vi "test_SetLogLevel_SetDebug_EventLogged.vi"(8 "error in (no error)":errorcluster, 11 "TestCase in":refnum<class "TestDataSink.lvclass">) -> (0 "error out":errorcluster, 3 "TestCase out":refnum<class "TestDataSink.lvclass">)   [LabVIEW 2017, in "TestDataSink.lvclass"]
uses:
  TestDataSink.lvclass
  Source/Composed Log/Types/Log Level.ctl
  Source/LVQueue Sink/LVQueue Sink.lvclass/LVQueue Sink.ctl
  Source/Composed Log/LoggerReference/LoggerReference.lvclass/LoggerReference.ctl
  Source/Composed Log/Log Sink/Log Sink.lvclass/Log Sink.ctl
  7e94cd01-c0ee-42ed-b087-4c2160652887.vi
  7e94cd01-c0ee-42ed-b087-4c2160652887.vi/e6a5d2d2-facc-43d0-9f34-28763a163c9b.vi
  Source/Composed Log/LoggerReference/Return Aggregate Queues.vi
  Source/Composed Log/LoggerReference/Add Aggregate Log.vi
  7e94cd01-c0ee-42ed-b087-4c2160652887.vi/e6a5d2d2-facc-43d0-9f34-28763a163c9b.vi/21c004db-7efd-4755-bf90-e0fdfa4dea43.vi
  Source/Composed Log/LoggerReference/Log.vi
  Source/Composed Log/LoggerReference/Send Add Sink.vi
  Source/Composed Log/LoggerReference/Remove Stale Logs.vi
  Source/LVQueue Sink/LVQueue Sink.lvclass
  C:/CS/Internal/LabVIEW/Logger/Source/Composed Log/Log Sink/Log Sink.lvclass
  Source/Composed Log/Application Logger/Launch Worker Loop.vi
  Source/Composed Log/LoggerReference/Initialize Logger Instance.vi
  Source/Composed Log/Singleton Event Log/Logger Queue FGV.vi
  Source/Composed Log/IErrorFormat/IErrorFormat.lvclass
  Source/Composed Log/LoggerReference/LoggerReference.lvclass
  Source/Composed Log/Log Sink/Log Sink.lvclass
  <vilib>/addons/_JKI Toolkits/VI Tester/TestCase.llb/TestCase.lvclass
  Source/Composed Log/Singleton Event Log/Singleton Event Log.lvlib
  Source/Composed Log/Composed Log.lvlib
  C:/Program Files (x86)/National Instruments/LabVIEW 2017/vi.lib/addons/_JKI Toolkits/VI Tester/TestCase.llb/TestCase.lvclass
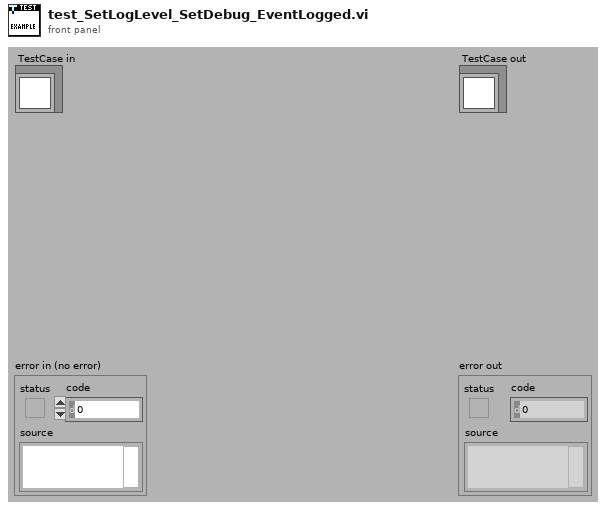
[diagram p1: front panel]
types:
  T1 = typedef "Composed Log.lvlib/Log Level.ctl" = enum16{"Debug", "Info", "Warning", "Error", "Critical"}
  T2 = typedef "Composed Log.lvlib/Log Packet.ctl" = cluster{"Data To Log":string, "Source":string, "Event Level":T1, "Event Time":timestamp}
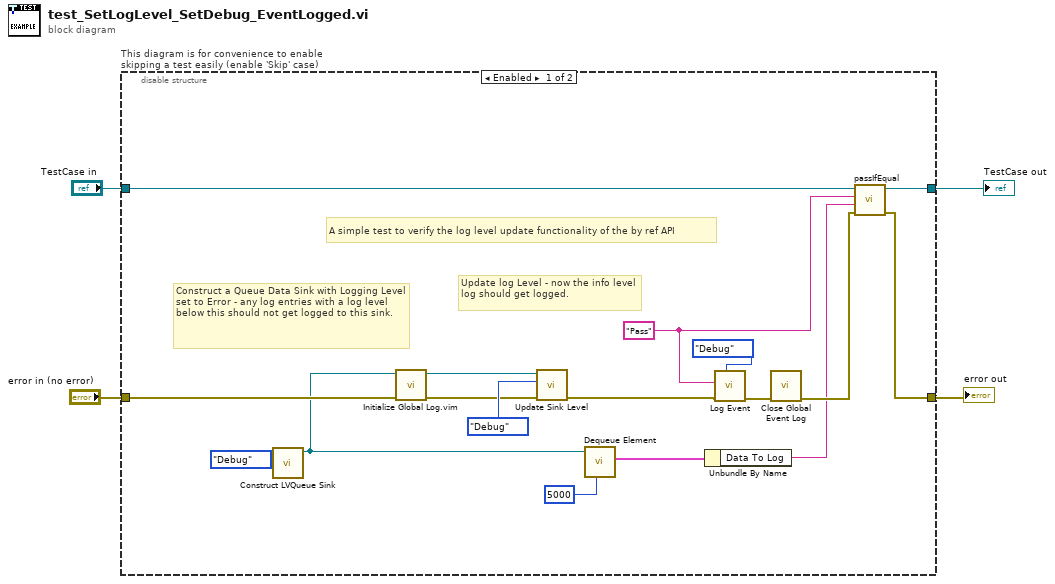
[diagram p0: block diagram]
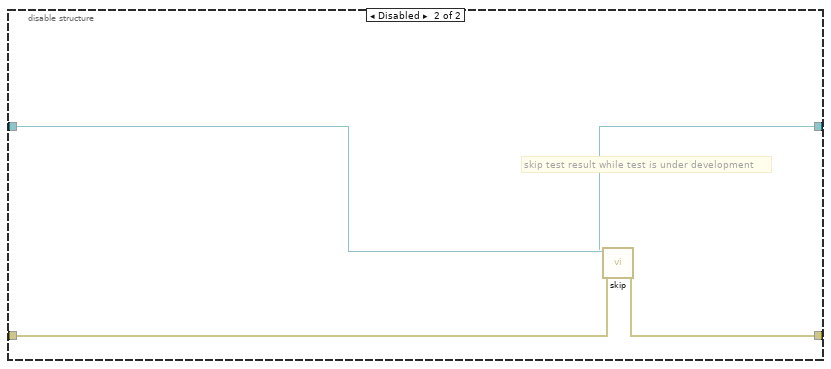
[diagram p2: hidden frame]
diagram:
  n1 = disable-structure "This diagram is for convenience to enable skipping a test easily (enable 'Skip' case)" shown="Enabled" {
    disable-tunnel: "TestCase in" -> [w18 w25]
    disable-tunnel: [w20 w23] -> w1
    disable-tunnel: [w19 w24] -> w3
    disable-tunnel: "error in (no error)" -> [w21 w22]
    frame Enabled {
      w6 = "Pass" ("Data To Log")
      # "Update log Level - now the info level log should get logged."
      # "A simple test to verify the log level update functionality of the by ref API"
      # "Construct a Queue Data Sink with Logging Level set to Error - any log entries with a log level below this should not get logged to this sink."
      n2 = call "Construct LVQueue Sink.vi"("LogLevel"=Log_Level."Debug") -> ("LVQueue Sink out"=w17:refnum<class "LVQueue Sink.lvclass">)  [unwired: 9 in, 1 out]
      n3 = call "Initialize Global Log.vim"("error in (no error)"=w21, "Log Sink(s)"=w17) -> ("error out"=w9:errorcluster, "Log Sink Reference(s)"=w15:refnum<data-value>)  [unwired: 8 in]
      n4 = call "Update Sink Level.vi"("error in (no error)"=w9, "LogLevel"=Log_Level."Debug", "Log Sink"=w15) -> ("error out"=w8:errorcluster)  [unwired: 8 in]
      n5 = call "Dequeue Element.vi"("timeout in ms (-1)"=5000, "LVQueue Sink in"=w17) -> ("Log Packet"=w12:T2)  [unwired: 6 in, 3 out]
      n6 = Unbundle By Name(w12) -> ("Data To Log"=w11:string)
      n7 = call "Log Event.vi"("Event Level"=Log_Level."Debug", "error in (no error)"=w8, "Data To Log"=w6) -> ("error out"=w7:errorcluster)  [unwired: 8 in]
      n8 = call "Close Global Event Log.vi"("error in (no error)"=w7) -> ("error out"=w13:errorcluster)  [unwired: 10 in]
      n9 = call-dynamic "passIfEqual.vi"("error in (no error)"=w13, "y"=w11, "x"=w6, "TestCase in"=w18) -> ("error out"=w19:errorcluster, "TestCase out"=w20:refnum<class "TestDataSink.lvclass">)  [unwired: 6 in]
    }
    frame Disabled {
      # "skip test result while test is under development"
      n10 = call <vilib>:"skip.vi"("error in (no error)"=w22, "TestCase in"=w25) -> ("error out"=w24:errorcluster, "TestCase out"=w23:refnum<class "TestDataSink.lvclass">)  [unwired: 8 in]
    }
  }
  "error out" <- w3
  "TestCase out" <- w1
